vi "boolean_function.vi"() -> ()   [LabVIEW 2019]
panel:
  out ".not. (x .xor. y)?":bool
  out "x .xor. y?":bool
  out "NAND":bool
  out "NOR":bool
  in  "input2":bool
  in  "input1 2":bool
  in  "input2":bool
  in  "input1":bool
  out "AND OR":bool
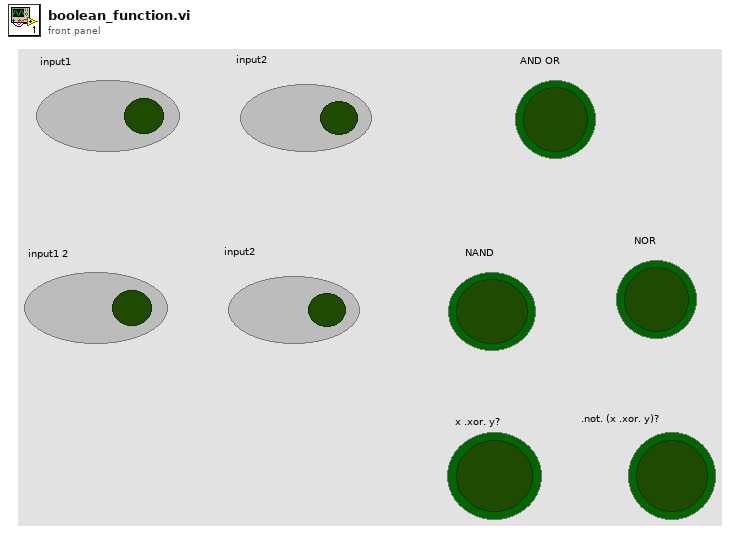
[diagram p1: front panel]
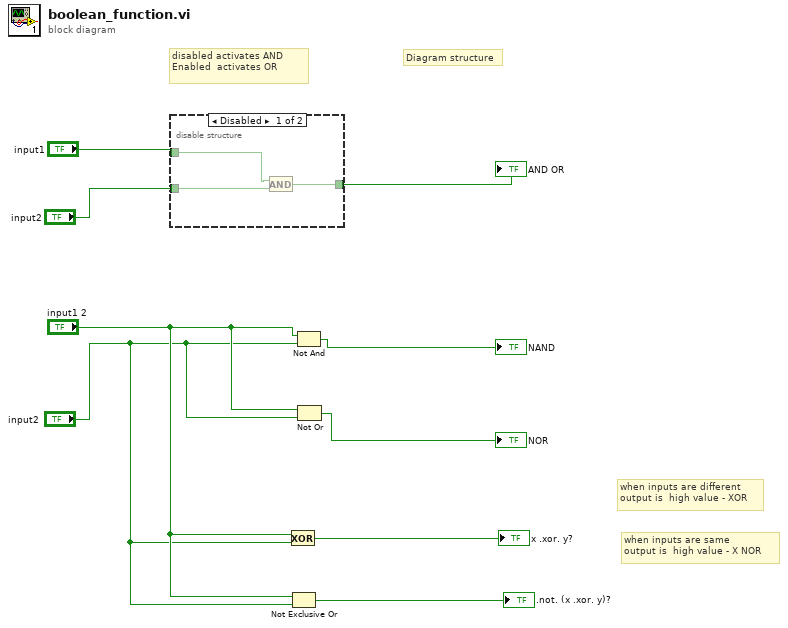
[diagram p0: block diagram]
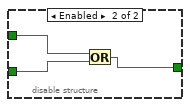
[diagram p2: hidden frame]
diagram:
  # "when inputs are same \noutput is  high value - X NOR"
  # "when inputs are different \noutput is  high value - XOR"
  # "Diagram structure"
  # "disabled activates AND\nEnabled  activates OR"
  n1 = disable-structure shown="Disabled" {
    disable-tunnel: "input2" -> [w12 w14]
    disable-tunnel: "input1" -> [w11 w15]
    disable-tunnel: [w10 w13] -> w9
    frame Disabled {
      n2 = And(x=w11, y=w12) -> (x .and. y?=w10:bool)
    }
    frame Enabled {
      n3 = Or(x=w15, y=w14) -> (x .or. y?=w13:bool)
    }
  }
  "AND OR" <- w9
  n4 = Exclusive Or(1:"input2", 2:"input1 2") -> (0:→"x .xor. y?":bool)
  n5 = Not Exclusive Or(1:"input2", 2:"input1 2") -> (0:→".not. (x .xor. y)?":bool)
  n6 = Not And(1:"input2", 2:"input1 2") -> (0:→"NAND":bool)
  n7 = Not Or(1:"input2", 2:"input1 2") -> (0:→"NOR":bool)
